vi "01AMT800_RAMPRES.vi"(4 "RES DOWN":bool, 5 "RES UP":bool, 6 "RAMP DOWN":bool, 7 "RAMP UP":bool, 8 "error in (no error)":errorcluster, 11 "Enum":enum16{"Initialize", "Set"}(ring)) -> (0 "error out":errorcluster, 2 "RAMP":dbl, 3 "RES":dbl)   [LabVIEW 2015]
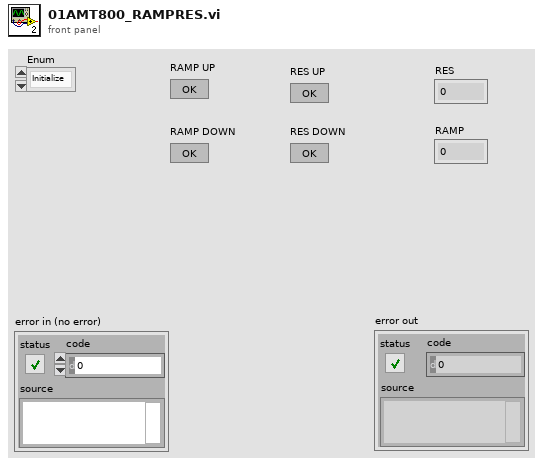
[diagram p1: front panel]
types:
  T1 = enum16{"Initialize", "Next", "Send RSET", "Set MPH", "Set INC", "Part to 0", "Get MPH", "Set RES", "Set RAMP"}
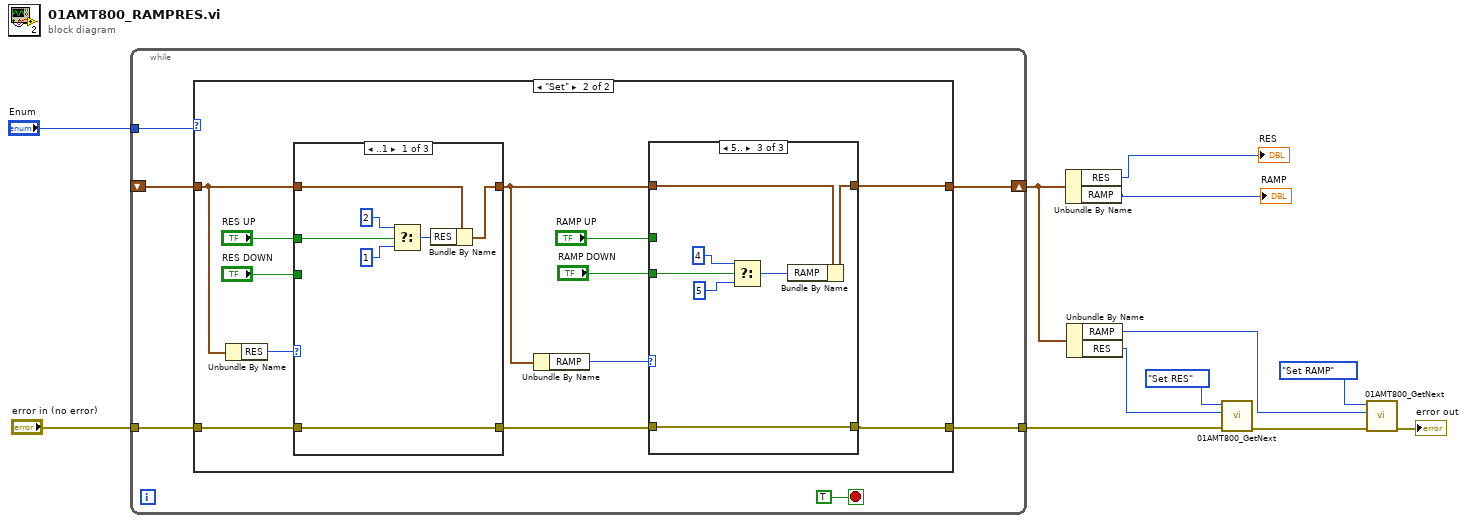
[diagram p0: block diagram]
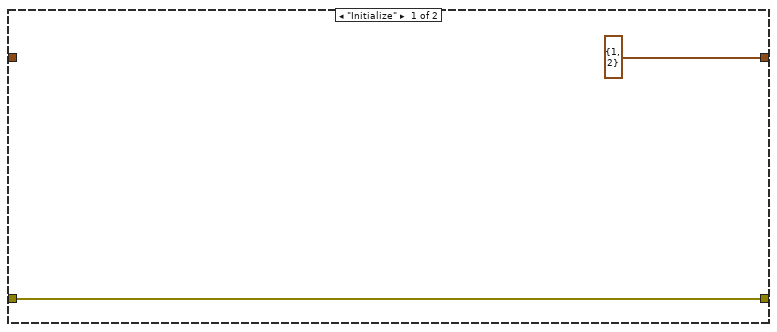
[diagram p2: hidden frame]
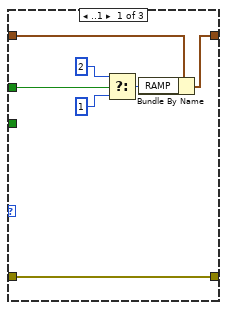
[diagram p3: hidden frame]
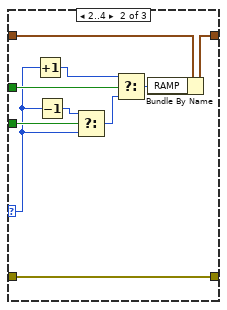
[diagram p4: hidden frame]
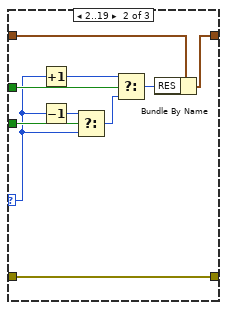
[diagram p5: hidden frame]
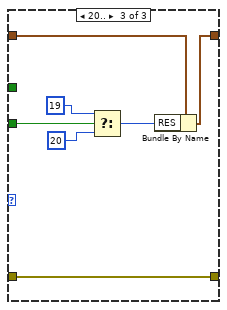
[diagram p6: hidden frame]
diagram:
  n1 = while {
    tunnel: "error in (no error)" -> [w17]
    tunnel: [w16] -> w8
    tunnel: "Enum" -> [w15]
    shift-right: [w14] -> w10
    shift-left: _ -> [w13]
    stop <- TRUE stop-if-true
    n2 = case shown="\"Set\"" w15 {
      tunnel: w17 -> [w20 w32]
      tunnel: [w20 w23] -> w16
      tunnel: [cluster{"RES":i32, "RAMP":i32} {"RES"=1, "RAMP"=2} w22] -> w14
      tunnel: w13 -> [_ w30]
      frame "Initialize" {
      }
      frame "Set" {
        n3 = Unbundle By Name(w30) -> ("RES"=w31:i32)
        n4 = case shown="..1" w31 {
          selector: w31 -> [_ w65 _]
          tunnel: w32 -> [w63 w73 w80]
          tunnel: [w63 w73 w80] -> w27
          tunnel: w30 -> [w61 w71 w78]
          tunnel: "RES UP" -> [w60 w70 _]
          tunnel: "RES DOWN" -> [_ w67 w77]
          tunnel: [w62 w72 w79] -> w26
          frame ..1 {
            n5 = Select(t=2 ("MPH"), s=w60, f=1 ("MPH")) -> (s? t:f=w59:i32)
            n6 = Bundle By Name(cluster=w61, "RES"=w59) -> (w62:cluster{"RES":i32, "RAMP":i32})
          }
          frame 2..19 {
            n7 = Increment(x=w65) -> (x+1=w64:i32)
            n8 = Decrement(x=w65) -> (x-1=w66:i32)
            n9 = Select(t=w66, s=w67, f=w65) -> (s? t:f=w68:i32)
            n10 = Select(t=w64, s=w70, f=w68) -> (s? t:f=w69:i32)
            n11 = Bundle By Name(cluster=w71, "RES"=w69) -> (w72:cluster{"RES":i32, "RAMP":i32})
          }
          frame 20.. {
            n12 = Select(t=19 ("MPH"), s=w77, f=20) -> (s? t:f=w76:i32)
            n13 = Bundle By Name(cluster=w78, "RES"=w76) -> (w79:cluster{"RES":i32, "RAMP":i32})
          }
        }
        n14 = Unbundle By Name(w26) -> ("RAMP"=w21:i32)
        n15 = case shown="5.." w21 {
          selector: w21 -> [_ w40 _]
          tunnel: w27 -> [w39 w49 w56]
          tunnel: [w39 w49 w56] -> w23
          tunnel: w26 -> [w37 w47 w54]
          tunnel: "RAMP UP" -> [w36 w46 _]
          tunnel: "RAMP DOWN" -> [_ w43 w53]
          tunnel: [w38 w48 w55] -> w22
          frame ..1 {
            n16 = Select(t=2 ("MPH"), s=w36, f=1 ("MPH")) -> (s? t:f=w35:i32)
            n17 = Bundle By Name(cluster=w37, "RAMP"=w35) -> (w38:cluster{"RES":i32, "RAMP":i32})
          }
          frame 2..4 {
            n18 = Increment(x=w40) -> (x+1=w42:i32)
            n19 = Decrement(x=w40) -> (x-1=w41:i32)
            n20 = Select(t=w41, s=w43, f=w40) -> (s? t:f=w44:i32)
            n21 = Select(t=w42, s=w46, f=w44) -> (s? t:f=w45:i32)
            n22 = Bundle By Name(cluster=w47, "RAMP"=w45) -> (w48:cluster{"RES":i32, "RAMP":i32})
          }
          frame 5.. {
            n23 = Select(t=4 ("MPH"), s=w53, f=5) -> (s? t:f=w52:i32)
            n24 = Bundle By Name(cluster=w54, "RAMP"=w52) -> (w55:cluster{"RES":i32, "RAMP":i32})
          }
        }
      }
    }
  }
  n25 = Unbundle By Name(w10) -> ("RES"=→"RES":i32, "RAMP"=→"RAMP":i32)
  n26 = Unbundle By Name(w10) -> ("RAMP"=w5:i32, "RES"=w9:i32)
  n27 = call "01AMT800_GetNext.vi"("error in (no error)"=w8, "Value"=w9, "Enum"=T1."Set RES") -> ("error out"=w6:errorcluster)  [unwired: 7 in, 1 out]
  n28 = call "01AMT800_GetNext.vi"("error in (no error)"=w6, "Value"=w5, "Enum"=T1."Set RAMP") -> ("error out"=→"error out":errorcluster)  [unwired: 7 in, 1 out]
